vi "Write Test running.vi"(7 "Send any changes now? (F)":bool, 8 "error in (no error)":errorcluster, 10 "Test running":bool, 11 "Fiber Auto Collimation state data in":refnum<class "Fiber Auto Collimation state data.lvclass">) -> (0 "error out":errorcluster, 3 "Fiber Auto Collimation state data out":refnum<class "Fiber Auto Collimation state data.lvclass">)   [LabVIEW 2018, in "Fiber Auto Collimation state data.lvclass"]
doc: "A Boolean which should be set to True whenever a test is running, usually to disable a number of controls."
uses:
  Fiber Auto Collimation state data.lvclass
  Fiber Auto Collimation state data.lvclass/Fiber Auto Collimation state data.ctl
  Tracked state data.ctl
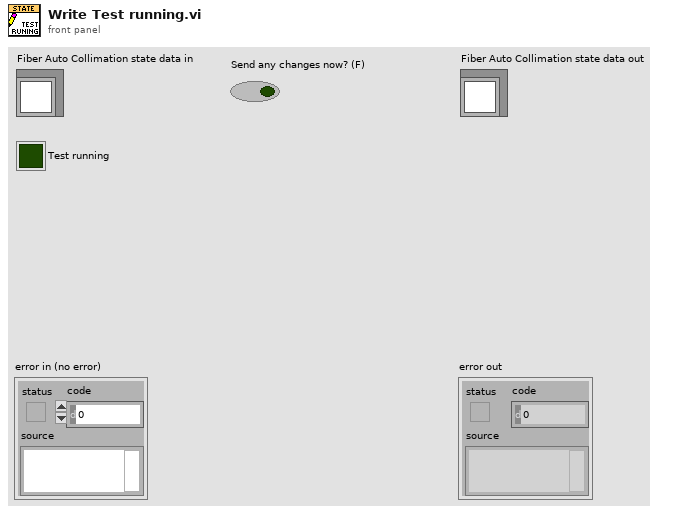
[diagram p1: front panel]
types:
  T1 = typedef "Fiber Auto Collimation state data.lvclass/Tracked state data.ctl" = enum16{"No update", "Permission level", "Username", "Test running", "DUT Serial", "Test status", "MOM Lot", "Loaded test recipe", "Model case running", "Station status", "BV data", "Defect Identify data", "Axis Position data", "Fiber Ass PN", "Operator", "RunTime", "VBAI", "Steps Cycle Time"}
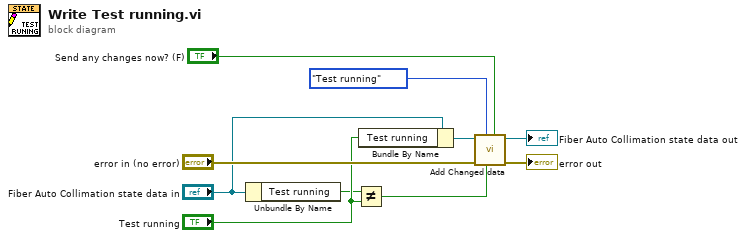
[diagram p0: block diagram]
diagram:
  n1 = Unbundle By Name("Fiber Auto Collimation state data in") -> ("Test running"=w2:bool)
  n2 = Not Equal?(x=w2, y="Test running") -> (x != y?=w3:bool)
  n3 = Bundle By Name(cluster="Fiber Auto Collimation state data in", "Test running"="Test running") -> (w6:refnum<class "Fiber Auto Collimation state data.lvclass">)
  n4 = call "Add Changed data.vi"("Send any changes now? (F)"="Send any changes now? (F)", "Data changed?"=w3, "Data type"=Tracked_state_data."Test running", "error in (no error)"="error in (no error)", "Fiber Auto Collimation state data in"=w6) -> ("error out"=→"error out":errorcluster, "Fiber Auto Collimation state data out"=→"Fiber Auto Collimation state data out":refnum<class "Fiber Auto Collimation state data.lvclass">)  [unwired: 5 in]
